vi "Song Library To Song Display.vi"(8 "error in (no error)":errorcluster, 11 "Song Library":refnum<class "SongLibrary.lvclass">) -> (0 "error out":errorcluster, 3 "Songs":T1[](array[typedef]) {"Duration (s)" format="%<%M:%S>T"})   [LabVIEW 2015, in "SongLibrary.lvclass"]
uses:
  SongLibrary.lvclass
  app/controls/Song Browser Display.ctl
  Song/Song Duration.ctl
  app/controls/Enqueue Control.ctl
  MusicElementLibrary.lvclass/MusicElementLibrary.ctl
  MusicElement.lvclass
  Song/Song.lvclass
  MusicElementLibrary.lvclass
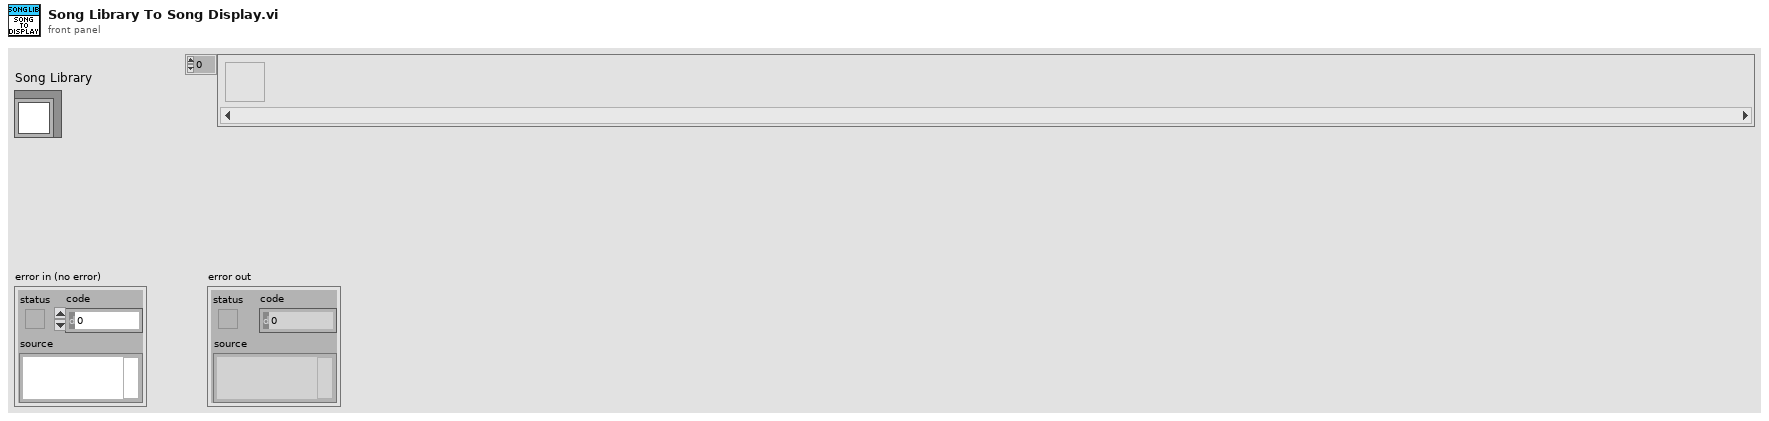
[diagram p1: front panel]
types:
  T1 = typedef "Song Browser Display.ctl" = cluster{"Song Name":string, "Artist":string, "Album":string, "Duration (s)":T2, "UID":string, "Enqueue":T3}
  T2 = typedef "Song.lvclass/Song Duration.ctl" = timestamp
  T3 = typedef "Enqueue Control.ctl" = bool
  T4 = typedef "Queue Song Display.ctl" = cluster{"Song Name":string, "Artist":string, "Album":string, "Duration (s)":T2, "UID":string, "Dequeue":T5}
  T5 = typedef "Dequeue Control.ctl" = bool
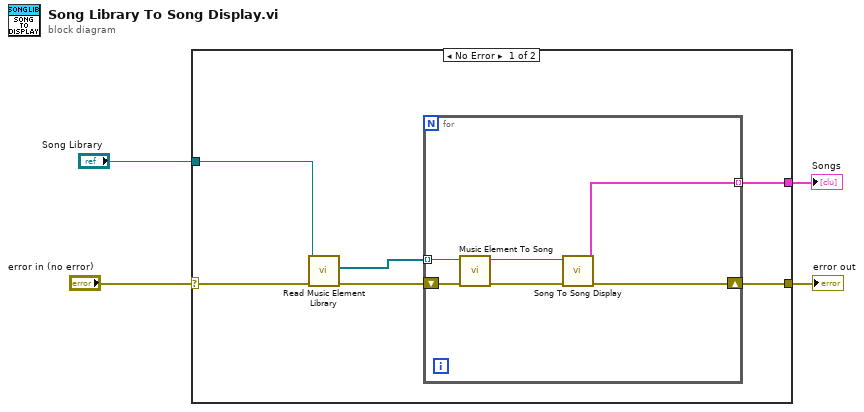
[diagram p0: block diagram]
diagram:
  n1 = case shown="No Error" "error in (no error)" {
    selector: "error in (no error)" -> [w8 w17]
    tunnel: [w10 w17] -> w3
    tunnel: "Song Library" -> [w6 _]
    tunnel: [w9 _] -> w1
    frame No Error {
      n2 = call "Read Music Element Library.vi"("error in (no error)"=w8, "MusicElementLibrary in"=w6) -> ("error out"=w7:errorcluster, "Music Element Library"=w5:refnum<class "MusicElement.lvclass">[])  [unwired: 7 in, 1 out]
      n3 = for {
        shift-right: [w16] -> w10
        shift-left: w7 -> [w14]
        tunnel: [w15] -> w9 mode=indexing
        tunnel: w5 -> [w12] mode=indexing
        n4 = call "Music Element To Song.vi"("error in (no error)"=w14, "MusicElement"=w12) -> ("error out"=w13:errorcluster, "Song out"=w11:refnum<class "Song.lvclass">)  [unwired: 8 in]
        n5 = call "Song To Song Display.vi"("error in (no error)"=w13, "Song"=w11) -> ("error out"=w16:errorcluster, "Song DIsplay"=w15:T4)  [unwired: 8 in]
      }
    }
    frame Error {
    }
  }
  "error out" <- w3
  "Songs" <- w1
